vi "Get Source Level.vi"(8 "error in (no error)":errorcluster, 11 "VISA resource name":refnum<visa-resource-name>) -> (0 "error out":errorcluster, 1 "Current Level Out":dbl, 2 "Voltage Level Out":dbl, 3 "VISA resource name out":refnum<visa-resource-name>)   [LabVIEW 2017, in "Keithley 2450.lvlib"]
doc: "This command returns the fixed amplitude for both the V & I source function."
uses:
  Keithley 2450.lvlib
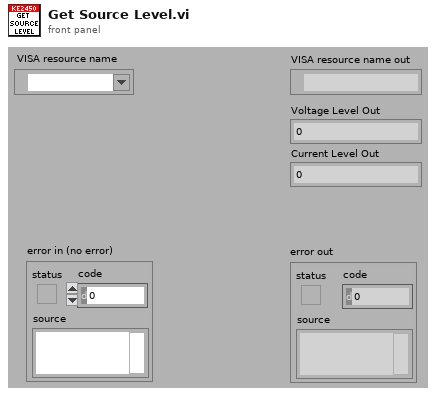
[diagram p1: front panel]
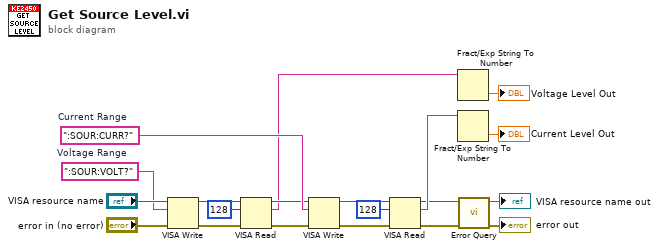
[diagram p0: block diagram]
diagram:
  w8 = ":SOUR:CURR?"  # Current Range
  w9 = ":SOUR:VOLT?"  # Voltage Range
  n1 = VISA Write(VISA resource name="VISA resource name", write buffer=w9, error in (no error)="error in (no error)") -> (VISA resource name out=w19:refnum<visa-resource-name>, error out=w20:errorcluster)  [unwired: 1 out]
  n2 = VISA Read(VISA resource name=w19, byte count=u32 128, error in (no error)=w20) -> (VISA resource name out=w7:refnum<visa-resource-name>, read buffer=w6:string, error out=w10:errorcluster)  [unwired: 1 out]
  n3 = VISA Write(VISA resource name=w7, write buffer=w8, error in (no error)=w10) -> (VISA resource name out=w12:refnum<visa-resource-name>, error out=w11:errorcluster)  [unwired: 1 out]
  n4 = VISA Read(VISA resource name=w12, byte count=u32 128, error in (no error)=w11) -> (VISA resource name out=w2:refnum<visa-resource-name>, read buffer=w5:string, error out=w1:errorcluster)  [unwired: 1 out]
  n5 = Fract/Exp String To Number(string=w6) -> (number=→"Voltage Level Out":dbl)  [unwired: 3 in, 1 out]
  n6 = Fract/Exp String To Number(string=w5) -> (number=→"Current Level Out":dbl)  [unwired: 3 in, 1 out]
  n7 = call "Error Query.vi"("error in (no error)"=w1, "VISA resource name"=w2) -> ("error out"=→"error out":errorcluster, "VISA resource name out"=→"VISA resource name out":refnum<visa-resource-name>)  [unwired: 8 out]
